vi "Noise_Analyse_1_Ch.vi"(5 "Test Parameters:":T5={"Temperature"=25.0, "Sampling Rate"=12800.0, "Coupling Mode"="DC"}, 7 "# of Averaging":u32=1, 11 "error in":errorcluster) -> (4 "Overall WriteData_Array":string[](array[string])=["114.527501913369", "0.000000083047", "10.600000000000", "0.000000365523", "114.596400074689", "0.000000082391", "12.600000000000", "0.000000348282", "114.703426082360", "0.000000081382", "4995.000000000000", "0.000000203014", "114.723850068193", "0.000000081191", "14.400000000000", "0.000000251425", "114.485379672127", "0.000000083451", "10.200000000000", "0.000000330843", "114.413402643394", "0.000000084145", "15.000000000000", "0.000000248333", "114.739058274487", "0.000000081049", "34.000000000000", "0.000000256843", "114.548482998097", "0.000000082847", "13.600000000000", "0.000000244620"], 15 "error out":errorcluster={"status"=FALSE, "code"=1906, "source"="SVFA Power Spectrum (1 Ch).vi:7340007"})   [LabVIEW 2018]
uses:
  <vilib>/addons/_NISVFA/_Shared subVIs/Controls/svc_Window.ctl
  <vilib>/Analysis/5stat.llb/RMS (DBL).vi
  <vilib>/addons/Sound and Vibration/svt_Single Tone Measurements/SVT Idle Channel Noise (Time) (1 Ch).vi
  <vilib>/addons/_NISVFA/_Baseband FFT/SVFA Power Spectral Density (1 Ch).vi
  <vilib>/addons/_NISVFA/_Baseband FFT/SVFA Power Spectrum (1 Ch).vi
  <vilib>/addons/Sound and Vibration/svt_Single Tone Measurements/SoundVib_SingleTone.lvlib
  <vilib>/Analysis/NI_AALBase.lvlib
  <vilib>/Analysis/NI_AALPro.lvlib
  <vilib>/gmath/NI_Gmath.lvlib
panel:
  out "CH0":cluster{"f0":dbl, "df":dbl, "magnitude":dbl[]}(graph)={"f0"=0.0, "df"=0.2, "magnitude"=[]}
  out "Graph_CH0":T1={"FFT Plot"={"f0"=0.0, "df"=0.2, "magnitude"=[]}, "Noise Density"={"f0"=0.0, "df"=0.2, "magnitude"=[]}, "Histogram"=[]}
  out "Data_CH0":T2={"SVT"={"Noise (BW)"=6.638588448604977e-06, "SNR [dB]"=114.52750191336867, "Avg Noise Density"=8.304726164455459e-08, "Maximum Spur"={"Frequency"=10.6, "Spur Level"=3.655230318410738e-07}}, "Max Data"=-9.28286463022232e-05, "Data Range"=6.53464812785387e-05, "Mean(Offset)"=-0.00012652362230801374, "StdDev (Noise)"=7.540583269192075e-06, "RMS Value"=0.00012674812231162398, "Spread Value"=0.0}
  in  "DUT Data":dbl[](array[numeric])
  out "dt":dbl=7.8125e-05
  out "frequency range":T3={"start frequency"=10.0, "stop frequency"=6400.0} {"stop frequency" format="%.2f"; "start frequency" format="%.2f"}
  out "DUT Data_CH0":dbl[](graph)
  out "averaging parameters":T4={"averaging mode"=enum."RMS averaging", "weighting mode"=enum."Linear", "number of averages"=1, "linear mode"=enum."Auto restart"} {"number of averages" min=1 step=1}
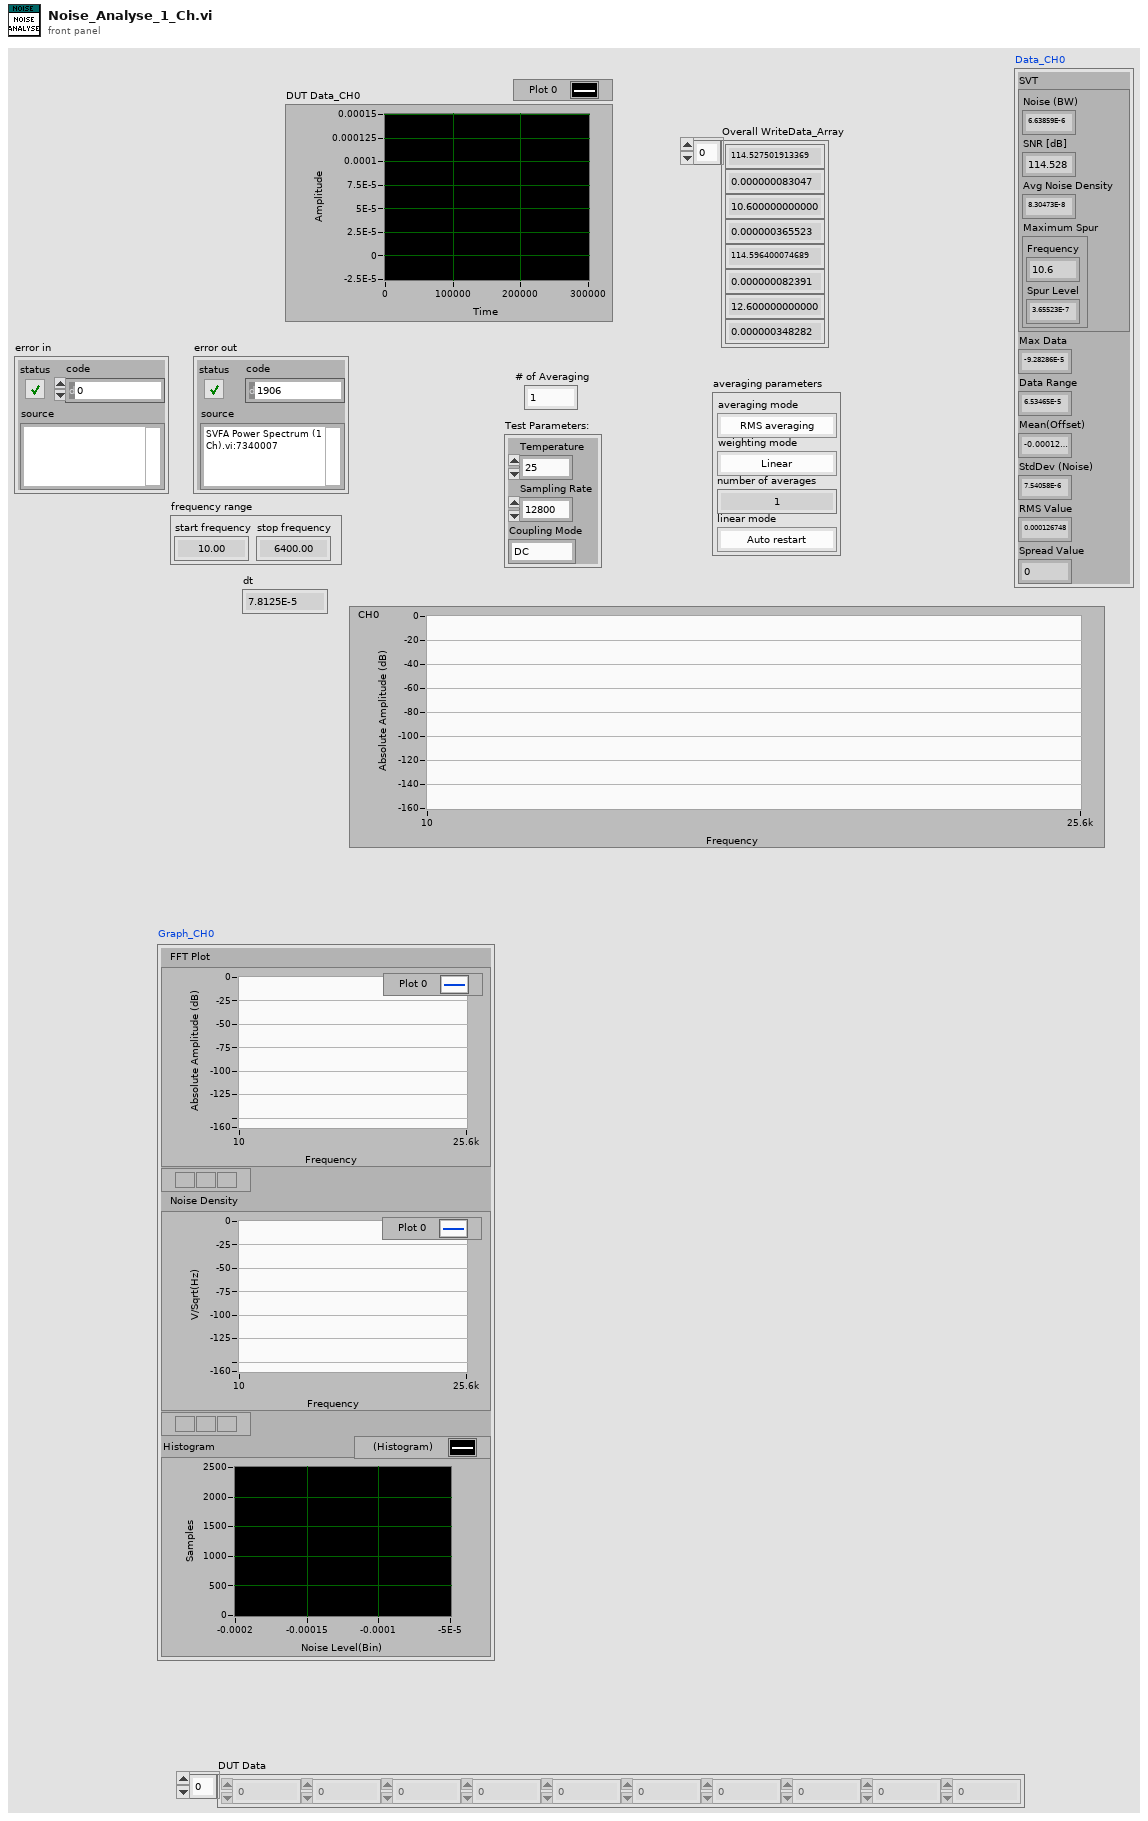
[diagram p1: front panel]
types:
  T1 = cluster{"FFT Plot":cluster{"f0":dbl, "df":dbl, "magnitude":dbl[]}, "Noise Density":cluster{"f0":dbl, "df":dbl, "magnitude":dbl[]}, "Histogram":dynamicdata}
  T2 = cluster{"SVT":cluster{"Noise (BW)":dbl, "SNR [dB]":dbl, "Avg Noise Density":dbl, "Maximum Spur":cluster{"Frequency":dbl, "Spur Level":dbl}}, "Max Data":dbl, "Data Range":dbl, "Mean(Offset)":dbl, "StdDev (Noise)":dbl, "RMS Value":dbl, "Spread Value":dbl}
  T3 = cluster{"start frequency":dbl, "stop frequency":dbl}
  T4 = cluster{"averaging mode":enum16{"No averaging", "Vector averaging", "RMS averaging", "Peak hold"}, "weighting mode":enum16{"Linear", "Exponential"}, "number of averages":u32, "linear mode":enum16{"One shot", "Auto restart"}}
  T5 = cluster{"Temperature":dbl, "Sampling Rate":dbl, "Coupling Mode":string}
  T6 = enum16{"No averaging", "Vector averaging", "RMS averaging", "Peak hold"}
  T7 = cluster{"idle channel noise units":enum16{"dB", "EU^2 rms"}}
  T8 = cluster{"Data_CH0":cluster{"SVT":cluster{"Noise (BW)":dbl, "SNR [dB]":dbl, "Avg Noise Density":dbl, "Maximum Spur":cluster{"Frequency":dbl, "Spur Level":dbl}}, "Max Data":dbl, "Data Range":dbl, "Mean(Offset)":dbl, "StdDev (Noise)":dbl, "RMS Value":dbl, "Spread Value":dbl}}
  T9 = typedef "svc_Window.ctl" = u32
  T10 = cluster{dbl, "SNR [dB]":dbl, "average noise level [EU / sqrt(Hz)]":dbl, "maximum spur [EU rms]":cluster{"frequency":dbl, "value":dbl}}
  T11 = cluster{cluster{dbl, "SNR [dB]":dbl, "average noise level [EU / sqrt(Hz)]":dbl, "maximum spur [EU rms]":cluster{"frequency":dbl, "value":dbl}}, dbl, dbl, "mean":dbl, "standard deviation":dbl, "rms value":dbl, "spread value":dbl}
  T12 = cluster{"power spectrum [dB EU]":cluster{"f0":dbl, "df":dbl, "magnitude":dbl[]}, "power spectral density [EU^2 rms / Hz]":cluster{"f0":dbl, "df":dbl, "magnitude":dbl[]}, "Histogram":dynamicdata}
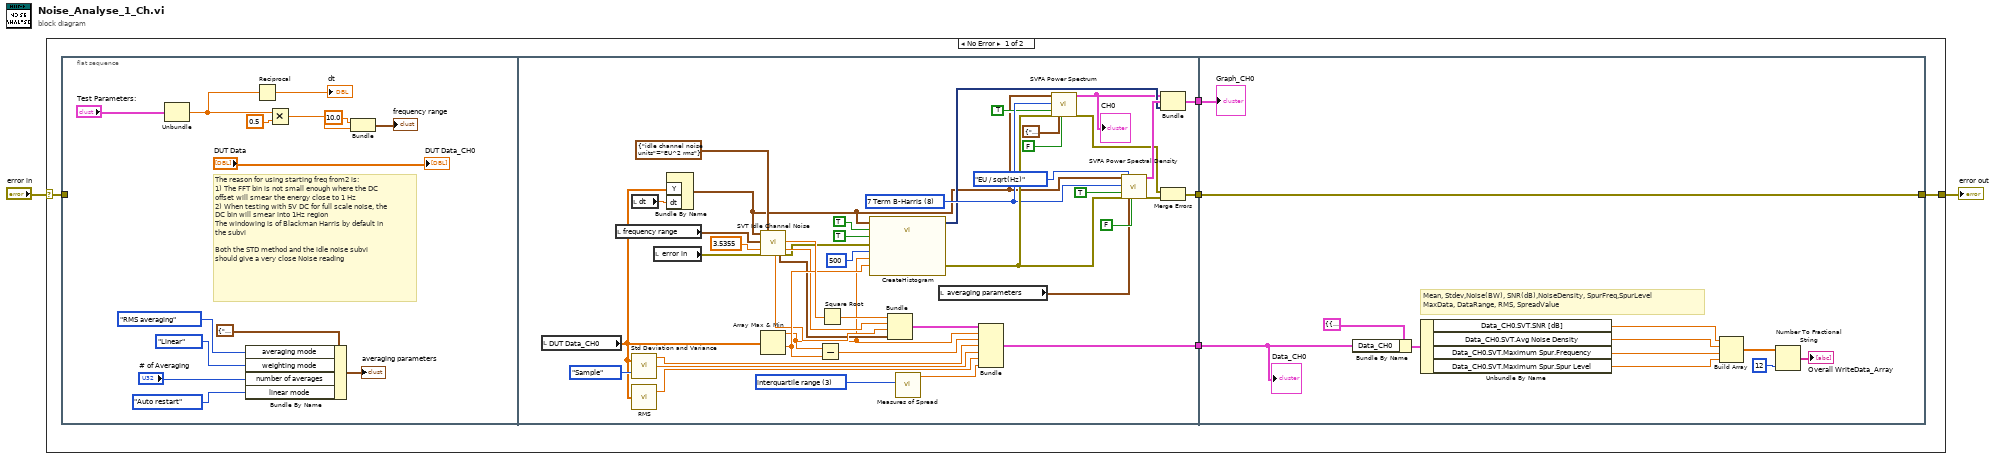
[diagram p0: block diagram]
diagram:
  n1 = case shown="No Error" "error in" {
    selector: "error in" -> [w3 w77]
    tunnel: [w4 w77] -> w2
    frame No Error {
      n2 = flat-sequence {
        tunnel: w3 -> [_]
        tunnel: [w29] -> w7
        tunnel: [w28] -> w6
        tunnel: [w24] -> w5
        tunnel: w7 -> [w69]
        tunnel: w6 -> [w74]
        tunnel: w5 -> [w72]
        tunnel: [w72] -> w4
        frame #0 {
          # "The reason for using starting freq from2 is:\n1) The FFT bin is not small enough where the DC offset will smear the energy close to 1 Hz\n2) When testing with 5V DC for full scale noise, the DC bin will smear into 1Hz region\nThe windowing is of Blackman Harris by default in the subvi\n\nBoth the STD method and the idle noise subvi should give a very close Noise reading"
          n3 = Unbundle("Test Parameters:") -> ("Sampling Rate"=w18:dbl)  [unwired: 2 out]
          n4 = Bundle By Name(cluster=T4 {"averaging mode"=enum."No averaging", "weighting mode"=enum."Exponential", "number of averages"=10, "linear mode"=enum."One shot"} ("averaging parameters"), "averaging mode"=T6."RMS averaging", "weighting mode"=enum16{"Linear", "Exponential"}."Linear", "number of averages"="# of Averaging", "linear mode"=enum16{"One shot", "Auto restart"}."Auto restart") -> (→"averaging parameters":T4)
          n5 = Reciprocal(x=w18) -> (1/x=→"dt":dbl)
          n6 = Multiply(x=w18, y=0.5) -> (x*y=w21:dbl)
          n7 = Bundle(10.0, w21) -> (→"frequency range":cluster{dbl, dbl})  [unwired: 1 in]
          "DUT Data_CH0" <- "DUT Data"
        }
        frame #1 {
          w42 = T9 8 items=["None"=0, "Hanning"=1, "Hamming"=2, "Blackman-Harris"=3, "Exact Blackman"=4, "Blackman"=5, "Flat Top"=6, "4 Term B-Harris "=7, "7 Term B-Harris"=8, "Low Sidelobe"=9, "Force"=64, "Exponential"=65, "Blackman Nuttall"=11, "Triangle"=30, "Bartlett-Hanning"=31, "Bohman"=32, "Parzen"=33, "Welch"=34, "Kaiser"=60, "Dolph-Chebyshev"=61, "Gaussian"=62] ("window")
          w57 = 3 items=["standard deviation", "range", "mean absolute deviation", "interquartile range"] ("type")
          n8 = local read "DUT Data_CH0"() -> (w27:dbl[])
          n9 = local read "frequency range"() -> (w32:T3)
          n10 = local read "dt"() -> (w33:dbl)
          n11 = call <vilib>:"Std Deviation and Variance.vi"("X"=w27, "Weighting (Sample)"=enum16{"Sample", "Population"}."Sample") -> ("mean"=w49:dbl, "standard deviation"=w48:dbl)  [unwired: 1 out]
          n12 = call-poly <vilib>:"RMS.vi"("X"=w27) -> ("rms value"=w47:dbl)  [unwired: 1 out]
          n13 = local read "error in"() -> (w30:errorcluster)
          n14 = Bundle By Name("Y"=w27, "dt"=w33) -> (w34:waveform(dbl))  [unwired: 1 in]
          n15 = call-poly <vilib>:"SVT Idle Channel Noise.vi"("scaled signal [EU]"=w34, "frequency range"=w32, "full-scale level [EU rms]"=3.5355, "error in (no error)"=w30, "desired units"=T7 {"idle channel noise units"=enum."EU^2 rms"}) -> ("average noise level [EU / sqrt(Hz)]"=w53:dbl, "maximum spur [EU rms]"=w52:cluster{"frequency":dbl, "value":dbl}, "idle channel noise"=w59:dbl, "SNR [dB]"=w54:dbl, "error out"=w45:errorcluster)  [unwired: 7 in, 3 out]
          n16 = Array Max & Min(array=w27) -> (max value=w51:dbl, min value=w56:dbl)  [unwired: 2 out]
          n17 = Subtract(x=w51, y=w56) -> (x-y=w50:dbl)
          n18 = Square Root(x=w59) -> (sqrt(x)=w55:dbl)
          n19 = call "CreateHistogram.vi"("Maximum Value"=w51, "Number of Bins"=500, "Minimum Value"=w56, "error in (no error)"=w45, "Reset"=TRUE, "Enable"=TRUE, "Signal"=w34) -> ("error out"=w43:errorcluster, "Histogram"=w35:dynamicdata)  [unwired: 3 in]
          n20 = Bundle(w55, "SNR [dB]"=w54, "average noise level [EU / sqrt(Hz)]"=w53, "maximum spur [EU rms]"=w52) -> (w22:T10)  [unwired: 1 in]
          n21 = call <vilib>:"Measures of Spread.vi"("type"=w57) -> ("spread value"=w46:dbl)  [unwired: 9 in, 1 out]
          n22 = local read "averaging parameters"() -> (w31:T4)
          n23 = Bundle(w22, w51, w50, "mean"=w49, "standard deviation"=w48, "rms value"=w47, "spread value"=w46) -> (w29:T11)  [unwired: 1 in]
          n24 = call-poly <vilib>:"SVFA Power Spectrum.vi"("scaled signal [EU]"=w34, "window"=w42, "dB On (T)"=TRUE, "error in (no error)"=w43, "averaging parameters"=T4 {"averaging mode"=enum."No averaging", "weighting mode"=enum."Exponential", "number of averages"=10, "linear mode"=enum."One shot"}, "restart averaging (F)"=FALSE) -> ("power spectrum [dB EU]"=w23:cluster{"f0":dbl, "df":dbl, "magnitude":dbl[]}, "error out"=w26:errorcluster)  [unwired: 8 in, 4 out]
          "CH0" <- w23
          n25 = call-poly <vilib>:"SVFA Power Spectral Density.vi"("scaled signal [EU]"=w34, "window"=w42, "dB On (F)"=TRUE, "error in (no error)"=w43, "desired units"=enum16{"EU^2 / Hz", "EU / sqrt(Hz)"}."EU / sqrt(Hz)", "averaging parameters"=w31, "restart averaging (F)"=FALSE) -> ("power spectral density [EU^2 rms / Hz]"=w36:cluster{"f0":dbl, "df":dbl, "magnitude":dbl[]}, "error out"=w25:errorcluster)  [unwired: 7 in, 4 out]
          n26 = Bundle("power spectrum [dB EU]"=w23, "power spectral density [EU^2 rms / Hz]"=w36, "Histogram"=w35) -> (w28:T12)  [unwired: 1 in]
          n27 = Merge Errors(w26, w25) -> (w24:errorcluster)
        }
        frame #2 {
          # "Mean, Stdev,Noise(BW), SNR(dB),NoiseDensity, SpurFreq,SpurLevel\nMaxData, DataRange, RMS, SpreadValue"
          n28 = Bundle By Name(cluster=T8 {"Data_CH0"={"SVT"={"Noise (BW)"=0.0, "SNR [dB]"=0.0, "Avg Noise Density"=0.0, "Maximum Spur"={"Frequency"=0.0, "Spur Level"=0.0}}, "Max Data"=0.0, "Data Range"=0.0, "Mean(Offset)"=0.0, "StdDev (Noise)"=0.0, "RMS Value"=0.0, "Spread Value"=0.0}} ("Overall Data"), "Data_CH0"=w69) -> (w70:T8)
          n29 = Unbundle By Name(w70) -> ("Data_CH0.SVT.SNR [dB]"=w68:dbl, "Data_CH0.SVT.Avg Noise Density"=w67:dbl, "Data_CH0.SVT.Maximum Spur.Frequency"=w66:dbl, "Data_CH0.SVT.Maximum Spur.Spur Level"=w65:dbl)
          n30 = Build Array(w68, w67, w66, w65) -> (w73:dbl[])
          n31 = Number To Fractional String(number=w73, precision (6)=i16 12) -> (F-format string=→"Overall WriteData_Array":string[])  [unwired: 2 in]
          "Data_CH0" <- w69
          "Graph_CH0" <- w74
        }
      }
    }
    frame Error {
    }
  }
  "error out" <- w2
